vi "Read ILC ADC Settings.vi"(8 "error in (no error)":errorcluster, 11 "Boot Loader in":refnum<class "Boot Loader.lvclass">) -> (0 "error out":errorcluster, 2 "ILC ADC Settings":T1={"Reference Voltage Vref"=0.0, "Nominal Input Range in Counts"=128, "Preamplifier Gain"=0, "Conversion Settling Cycles"=0} {"Conversion Settling Cycles" min=1; "Preamplifier Gain" min=1; "Nominal Input Range in Counts" min=128; "Reference Voltage Vref" min=-10.0 max=10.0 format="%.3f"}, 3 "Boot Loader out":refnum<class "Boot Loader.lvclass">)   [LabVIEW 2015, in "Boot Loader.lvclass"]
uses:
  Boot Loader.lvclass
  <userlib>/Common/ILC/Configuration/ADC.ctl
  Settings/Settings.lvclass
  <userlib>/Common/ILC/Configuration/ILCConfiguration.lvlib
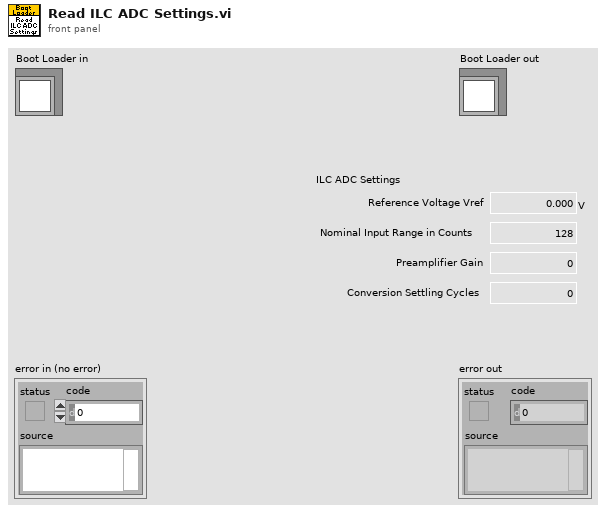
[diagram p1: front panel]
types:
  T1 = typedef "ILCCommon.lvlib/ILCConfiguration.lvlib/ADC.ctl" = cluster{"Reference Voltage Vref":dbl[unit], "Nominal Input Range in Counts":u32, "Preamplifier Gain":u8, "Conversion Settling Cycles":u16}
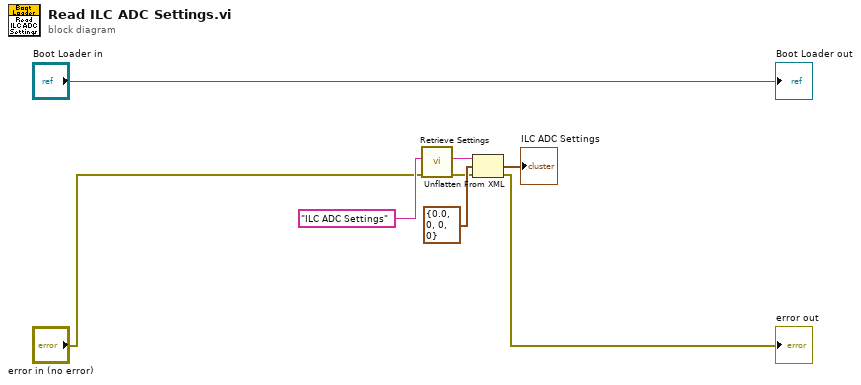
[diagram p0: block diagram]
diagram:
  n1 = call "Retrieve Settings.vi"("error in (no error)"="error in (no error)", "configName"="ILC ADC Settings") -> ("error out"=w3:errorcluster, "xmlConfig"=w6:string)  [unwired: 7 in, 1 out]
  n2 = Unflatten From XML(xml string=w6, type=T1 {"Reference Voltage Vref"=0.0, "Nominal Input Range in Counts"=0, "Preamplifier Gain"=0, "Conversion Settling Cycles"=0} ("ILC ADC"), error in (no error)=w3) -> (value=→"ILC ADC Settings":T1, error out=→"error out":errorcluster)
  "Boot Loader out" <- "Boot Loader in"
